vi "ToolStripItem.vi"(4 "Shortcut Keys":i32[](array[ring]) items=["None"=0, "LButton"=1, "RButton"=2, "Cancel"=3, "MButton"=4, "XButton1"=5, "XButton2"=6, "Back"=8, "Tab"=9, "LineFeed"=10, "Clear"=12, "Enter, Return"=13, "ShiftKey"=16, "ControlKey"=17, "Menu"=18, "Pause"=19, "CapsLock, Capital"=20, "HangulMode, HanguelMode, KanaMode"=21, "JunjaMode"=23, "FinalMode"=24, "KanjiMode, HanjaMode"=25, "Escape"=27, "IMEConvert"=28, "IMENonconvert"=29, "IMEAccept, IMEAceept"=30, "IMEModeChange"=31, "Space"=32, "Prior, PageUp"=33, "PageDown, Next"=34, "End"=35, "Home"=36, "Left"=37, "Up"=38, "Right"=39, "Down"=40, "Select"=41, "Print"=42, "Execute"=43, "Snapshot, PrintScreen"=44, "Insert"=45, "Delete"=46, "Help"=47, "D0"=48, "D1"=49, "D2"=50, "D3"=51, "D4"=52, "D5"=53, "D6"=54, "D7"=55, "D8"=56, "D9"=57, "A"=65, "B"=66, "C"=67, "D"=68, "E"=69, "F"=70, "G"=71, "H"=72, "I"=73, "J"=74, "K"=75, "L"=76, "M"=77, "N"=78, "O"=79, "P"=80, "Q"=81, "R"=82, "S"=83, "T"=84, "U"=85, "V"=86, "W"=87, "X"=88, "Y"=89, "Z"=90, "LWin"=91, "RWin"=92, "Apps"=93, "Sleep"=95, "NumPad0"=96, "NumPad1"=97, "NumPad2"=98, "NumPad3"=99, "NumPad4"=100, "NumPad5"=101, "NumPad6"=102, "NumPad7"=103, "NumPad8"=104, "NumPad9"=105, "Multiply"=106, "Add"=107, "Separator"=108, "Subtract"=109, "Decimal"=110, "Divide"=111, "F1"=112, "F2"=113, "F3"=114, "F4"=115, "F5"=116, "F6"=117, "F7"=118, "F8"=119, "F9"=120, "F10"=121, "F11"=122, "F12"=123, "F13"=124, "F14"=125, "F15"=126, "F16"=127, "F17"=128, "F18"=129, "F19"=130, "F20"=131, "F21"=132, "F22"=133, "F23"=134, "F24"=135, "NumLock"=144, "Scroll"=145, "LShiftKey"=160, "RShiftKey"=161, "LControlKey"=162, "RControlKey"=163, "LMenu"=164, "RMenu"=165, "BrowserBack"=166, "BrowserForward"=167, "BrowserRefresh"=168, "BrowserStop"=169, "BrowserSearch"=170, "BrowserFavorites"=171, "BrowserHome"=172, "VolumeMute"=173, "VolumeDown"=174, "VolumeUp"=175, "MediaNextTrack"=176, "MediaPreviousTrack"=177, "MediaStop"=178, "MediaPlayPause"=179, "LaunchMail"=180, "SelectMedia"=181, "LaunchApplication1"=182, "LaunchApplication2"=183, "OemSemicolon, Oem1"=186, "Oemplus"=187, "Oemcomma"=188, "OemMinus"=189, "OemPeriod"=190, "Oem2, OemQuestion"=191, "Oem3, Oemtilde"=192, "Oem4, OemOpenBrackets"=219, "OemPipe, Oem5"=220, "OemCloseBrackets, Oem6"=221, "OemQuotes, Oem7"=222, "Oem8"=223, "Oem102, OemBackslash"=226, "ProcessKey"=229, "Packet"=231, "Attn"=246, "Crsel"=247, "Exsel"=248, "EraseEof"=249, "Play"=250, "Zoom"=251, "NoName"=252, "Pa1"=253, "OemClear"=254, "KeyCode"=65535, "Shift"=65536, "Control"=131072, "Alt"=262144, "Modifiers"=-65536], 5 "ToolTip":string, 6 "Icon":path, 7 "SelectionType":refnum<class "MGI_SelectionType.lvclass">, 10 "error in (no error)":errorcluster, 11 "Text":string) -> (2 "error out":errorcluster, 3 "ToolStripItem":refnum<data-value>)   [LabVIEW 2019, in "MGI_ToolStripItem.lvclass"]
uses:
  MGI_ToolStripItem.lvclass
  <userlib>/_MGI/Menu Building/SelectionType/MGI_SelectionType.lvclass
  C:/Program Files (x86)/National Instruments/LabVIEW 2019/user.lib/_MGI/Menu Building/MenuItem/MGI_MenuItem.lvclass
  MGI_ToolStripItem.lvclass/MGI_ToolStripItem.ctl
  <userlib>/_MGI/Menu Building/MenuItem/MGI_MenuItem.lvclass
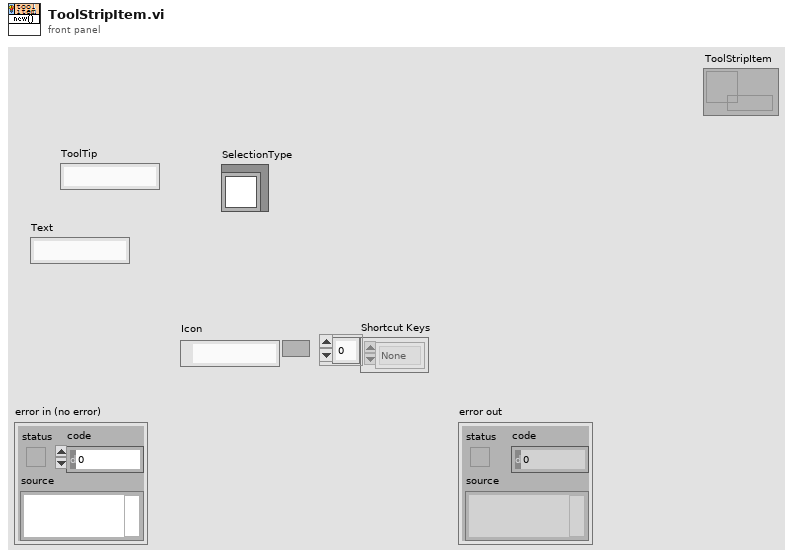
[diagram p1: front panel]
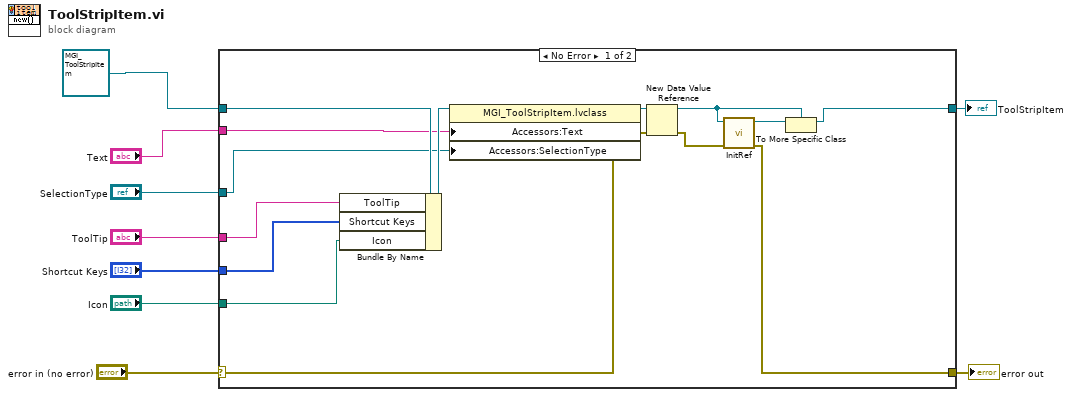
[diagram p0: block diagram]
diagram:
  n1 = case shown="No Error" "error in (no error)" {
    selector: "error in (no error)" -> [w19 w24]
    tunnel: [w10 w24] -> w8
    tunnel: [w12 _] -> w1
    tunnel: refnum<class "MGI_ToolStripItem.lvclass"> refnum ("MGI_ToolStripItem.lvclass") -> [w23 _]
    tunnel: "Text" -> [w20 _]
    tunnel: "ToolTip" -> [w18 _]
    tunnel: "Shortcut Keys" -> [w17 _]
    tunnel: "Icon" -> [w16 _]
    tunnel: "SelectionType" -> [w15 _]
    frame No Error {
      n2 = Bundle By Name(cluster=w23, "ToolTip"=w18, "Shortcut Keys"=w17, "Icon"=w16) -> (w22:refnum<class "MGI_ToolStripItem.lvclass">)
      n3 = property class="MGI_ToolStripItem.lvclass"(reference=w22, "Accessors:Text"=w20, "Accessors:SelectionType"=w15) -> (reference out=w21:refnum<class "MGI_ToolStripItem.lvclass">)  [unwired: 1 in, 1 out]
      n4 = New Data Value Reference(data value=w21, error in=w19) -> (data value reference=w13:refnum<data-value>, error out=w11:errorcluster)
      n5 = call <userlib>:"InitRef.vi"("error in (no error)"=w11, "MenuItem in"=w13) -> ("error out"=w10:errorcluster, "MenuItem out"=w14:refnum<data-value>)  [unwired: 8 in]
      n6 = To More Specific Class(target class=w13, reference=w14) -> (specific class reference=w12:refnum<data-value>)  [unwired: 1 in, 1 out]
    }
    frame Error {
    }
  }
  "error out" <- w8
  "ToolStripItem" <- w1
